vi "uActor_Get Self Transport (Community).vi"(11 "uActor in":refnum<class "uActor.lvclass">) -> (2 "Actor Transport":refnum<class "uTransport_uActor.lvclass">, 3 "uActor out":refnum<class "uActor.lvclass">)   [LabVIEW 2023, in "uLib.lvlib" / "uActor.lvclass"]
doc: "Wrapper for a protected method to expose to friend classes."
uses:
  uActor.lvclass
  uTransport/uTransport_uActor/uTransport_uActor.lvclass
  uActor.lvclass/uActor.ctl
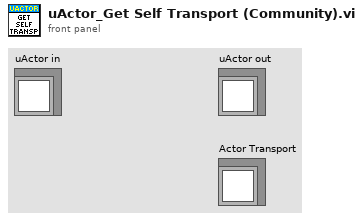
[diagram p1: front panel]
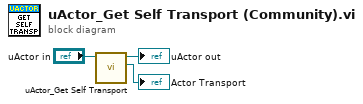
[diagram p0: block diagram]
diagram:
  n1 = call "uActor_Get Self Transport.vi"("uActor in"="uActor in") -> ("Actor Transport"=→"Actor Transport":refnum<class "uTransport_uActor.lvclass">, "uActor out"=→"uActor out":refnum<class "uActor.lvclass">)  [unwired: 9 in]
